vi "Launch XY Stage Class Proccess.vi"(8 "error in (no error)":errorcluster, 9 "Y Stage":refnum<class "iMotion Controller.lvclass">, 10 "X Stage":refnum<class "iMotion Controller.lvclass">, 11 "XY Stage Controller in":refnum<class "XY Stage Controller.lvclass">) -> (0 "error out":errorcluster, 3 "XY Stage Controller out":refnum<class "XY Stage Controller.lvclass">)   [LabVIEW 2022 SP3, in "XY Stage Process.lvlib" / "XY Stage Process.lvclass"]
uses:
  XY Stage Process.lvclass
  XY Stage Process.lvclass/XY Stage Process.ctl
  XY Stage Data Class/XY Stage Data Class.lvclass
  <vilib>/ActorFramework/Actor/Actor.lvclass
  XY Stage Controller/XY Stage Controller.lvclass
  Process Framework/Process State Data/Process State Data.lvclass
  Process Framework/Interlock Q Class/Interlock Q Class.lvclass
  C:/Program Files/National Instruments/LabVIEW 2022/vi.lib/ActorFramework/Actor/Actor.lvclass
  Axis Objects/iMotion Controller/iMotion Controller.lvclass
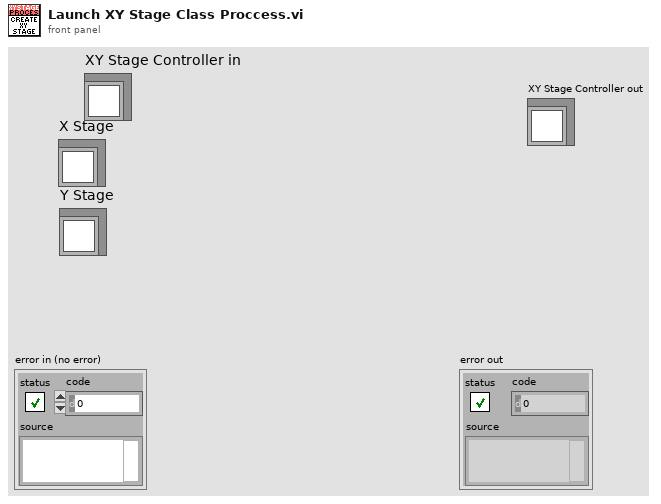
[diagram p1: front panel]
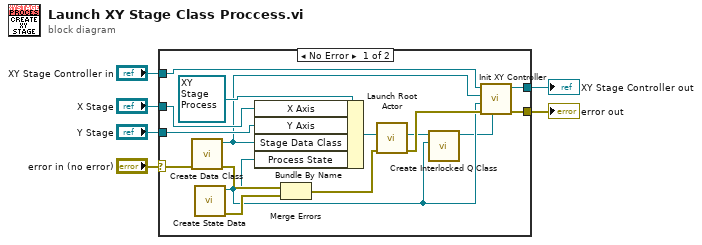
[diagram p0: block diagram]
diagram:
  n1 = case shown="No Error" "error in (no error)" {
    selector: "error in (no error)" -> [w17 w23]
    tunnel: [w13 w23] -> w5
    tunnel: "X Stage" -> [w21 _]
    tunnel: "Y Stage" -> [w20 _]
    tunnel: [w15 _] -> w2
    tunnel: "XY Stage Controller in" -> [w7 _]
    frame No Error {
      n2 = call "Create Data Class.vi"("error in (no error)"=w17) -> ("error out"=w16:errorcluster, "DVR"=w18:refnum<data-value>)  [unwired: 9 in]
      n3 = call "Create State Data.vi"() -> ("error out"=w11:errorcluster, "Process State Data out"=w10:refnum<data-value>)  [unwired: 10 in]
      n4 = Bundle By Name(cluster=refnum<class "XY Stage Process.lvclass"> refnum ("XY Stage Process in"), "X Axis"=w21, "Y Axis"=w20, "Stage Data Class"=w18, "Process State"=w10) -> (w19:refnum<class "XY Stage Process.lvclass">)
      n5 = Merge Errors(w16, w11) -> (w12:errorcluster)
      n6 = call <vilib>:"Launch Root Actor.vi"("error in (no error)"=w12, "Actor"=w19) -> ("error out"=w14:errorcluster, "Actor's Enqueuer"=w9:refnum<class "Message Enqueuer.lvclass">)  [unwired: 8 in]
      n7 = call "Create Interlocked Q Class.vi"("Process State Data"=w10, "Process Q"=w9) -> ("Interlock Q Class out"=w8:refnum<class "Interlock Q Class.lvclass">)  [unwired: 9 in]
      n8 = call "Init XY Controller.vi"("Interlock Q Class"=w8, "error in (no error)"=w14, "Process State Data"=w10, "Stage State Data"=w18, "XY Stage Controller"=w7) -> ("error out"=w13:errorcluster, "XY Stage Controller"=w15:refnum<class "XY Stage Controller.lvclass">)  [unwired: 5 in]
    }
    frame Error {
    }
  }
  "error out" <- w5
  "XY Stage Controller out" <- w2
